vi "Выбор subVI ПИД.vi"(10 "Array":dbl[](array[numeric]), 11 "Температура\nдома":dbl) -> (3 "Numeric":dbl)   [LabVIEW 2021]
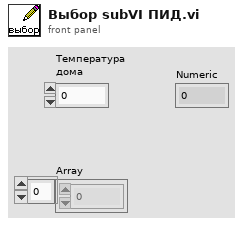
[diagram p1: front panel]
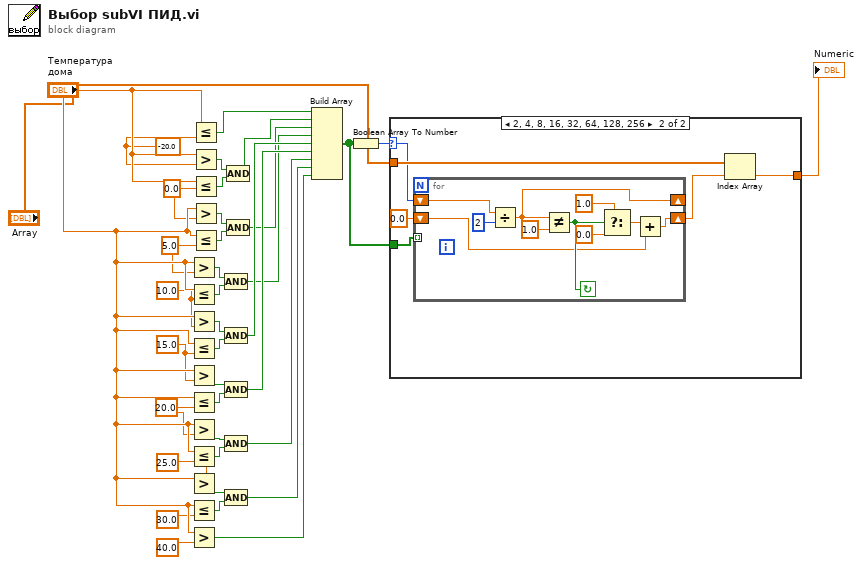
[diagram p0: block diagram]
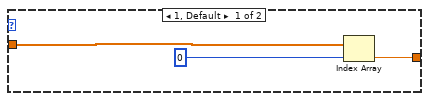
[diagram p2: hidden frame]
diagram:
  w25 = 25.0 ("y")
  w21 = 20.0 ("y")
  w18 = 15.0 ("y")
  w14 = 10.0 ("y")
  w12 = 5.0 ("y")
  w9 = 0.0 ("y")
  w8 = -20.0 ("y")
  n1 = Greater?(x="Температура\nдома", y=w12) -> (0:w11:bool)
  n2 = Less Or Equal?(x="Температура\nдома", y=w14) -> (x <= y?=w10:bool)
  n3 = Greater?(x="Температура\nдома", y=w14) -> (0:w15:bool)
  n4 = Less Or Equal?(x="Температура\nдома", y=w18) -> (x <= y?=w13:bool)
  n5 = Greater?(x="Температура\nдома", y=w18) -> (0:w17:bool)
  n6 = Less Or Equal?(x="Температура\nдома", y=w21) -> (x <= y?=w16:bool)
  n7 = Greater?(x="Температура\nдома", y=w21) -> (0:w19:bool)
  n8 = Less Or Equal?(x="Температура\nдома", y=w25) -> (x <= y?=w20:bool)
  n9 = Greater?(x="Температура\nдома", y=w25) -> (0:w24:bool)
  n10 = Less Or Equal?(x="Температура\nдома", y=30.0) -> (x <= y?=w23:bool)
  n11 = Greater?(x="Температура\nдома", y=40.0) -> (0:w33:bool)
  n12 = Less Or Equal?(x="Температура\nдома", y=w8) -> (x <= y?=w1:bool)
  n13 = Greater?(x="Температура\nдома", y=w8) -> (0:w4:bool)
  n14 = Less Or Equal?(x="Температура\nдома", y=w9) -> (x <= y?=w3:bool)
  n15 = Greater?(x="Температура\nдома", y=w9) -> (0:w6:bool)
  n16 = Less Or Equal?(x="Температура\nдома", y=w12) -> (x <= y?=w7:bool)
  n17 = Compound Arithmetic op=AND(w11, w10) -> (w28:bool)
  n18 = Compound Arithmetic op=AND(w15, w13) -> (w29:bool)
  n19 = Compound Arithmetic op=AND(w17, w16) -> (w30:bool)
  n20 = Compound Arithmetic op=AND(w19, w20) -> (w31:bool)
  n21 = Compound Arithmetic op=AND(w24, w23) -> (w32:bool)
  n22 = Compound Arithmetic op=AND(w4, w3) -> (w5:bool)
  n23 = Compound Arithmetic op=AND(w6, w7) -> (w27:bool)
  n24 = Build Array(w1, w5, w27, w28, w29, w30, w31, w32, w33) -> (w35:bool[])
  n25 = Boolean Array To Number(Boolean array=w35) -> (number=w2:u32)
  n26 = case shown="2, 4, 8, 16, 32, 64, 128, 256" w2 {
    selector: w2 -> [_ w44]
    tunnel: "Array" -> [w40 w46]
    tunnel: [w38 w45] -> w36
    tunnel: w35 -> [_ w41]
    frame 1, Default {
      n27 = Index Array(array=w40, index=0) -> (element=w38:dbl)
    }
    frame 2, 4, 8, 16, 32, 64, 128, 256 {
      n28 = for {
        shift-right: [w53] -> _
        shift-left: w44 -> [w56]
        shift-right: [w47] -> w42
        shift-left: 0.0 -> [w48]
        tunnel: w41 -> [_] mode=indexing
        stop <- w51 continue-if-true
        n29 = Divide(x=w56, y=u32 2) -> (x/y=w53:dbl)
        n30 = Not Equal?(x=w53, y=1.0) -> (x != y?=w51:bool)
        n31 = Select(t=1.0 ("y"), s=w51, f=0.0) -> (s? t:f=w49:dbl)
        n32 = Add(x=w49, y=w48) -> (x+y=w47:dbl)
      }
      n33 = Index Array(array=w46, index=w42) -> (element=w45:dbl)
    }
  }
  "Numeric" <- w36
